vi "Read Server Generic UE.vi"(11 "Template Server in":refnum<class "Streamer_server.lvclass">) -> (2 "Server Generic UE":refnum<user-event>, 3 "Template Server out":refnum<class "Streamer_server.lvclass">)   [LabVIEW 2019, in "Streamer_server.lvlib" / "Streamer_server.lvclass"]
uses:
  Streamer_server.lvclass
  <vilib>/gRPC/LabVIEW gRPC Library/Server API/typeDefs/Generic Method Event Data.ctl
  <vilib>/gRPC/LabVIEW gRPC Library/Server API/typeDefs/grpcId.ctl
  Streamer_server.lvclass/Streamer_server.ctl
  <vilib>/gRPC/LabVIEW gRPC Library/gprc-lvsupport-release.lvlib
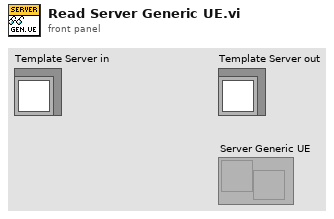
[diagram p1: front panel]
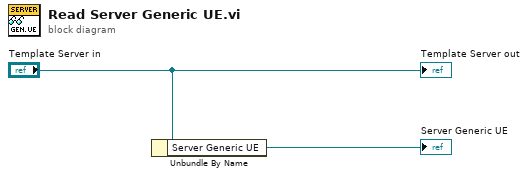
[diagram p0: block diagram]
diagram:
  n1 = Unbundle By Name("Template Server in") -> ("Server Generic UE"=→"Server Generic UE":refnum<user-event>)
  "Template Server out" <- "Template Server in"
